vi "from string 1.0.vi"(8 "error in":errorcluster, 10 "data in":string, 11 "Shared Memory configuration in":refnum<class "Shared Memory configuration.lvclass">) -> (0 "error out":errorcluster, 2 "remaining data":string, 3 "Shared Memory configuration out":refnum<class "Shared Memory configuration.lvclass">)   [LabVIEW 2014, in "Shared Memory configuration.lvclass"]
uses:
  Shared Memory configuration.lvclass
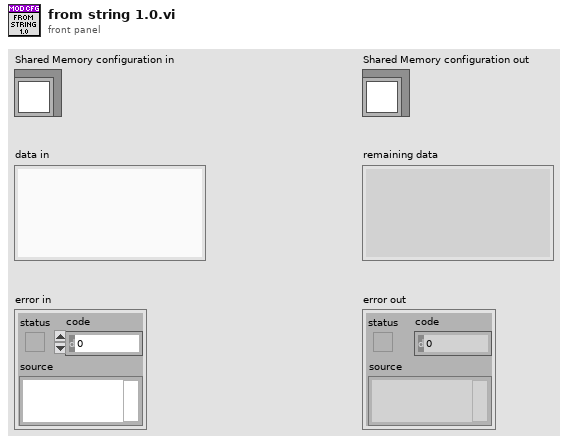
[diagram p1: front panel]
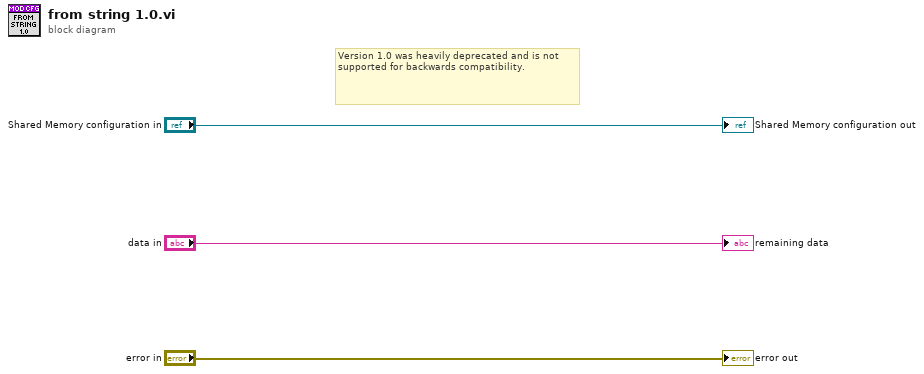
[diagram p0: block diagram]
diagram:
  # "Version 1.0 was heavily deprecated and is not supported for backwards compatibility."
  "error out" <- "error in"
  "Shared Memory configuration out" <- "Shared Memory configuration in"
  "remaining data" <- "data in"
